vi "Close Private.vi"(8 "error in (no error)":errorcluster) -> (0 "error out":errorcluster)   [LabVIEW 2020, in "Better Search.lvlib" / "BetterSearch.lvclass"]
uses:
  BetterSearch.lvclass
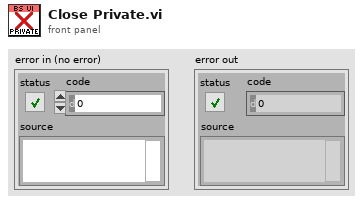
[diagram p1: front panel]
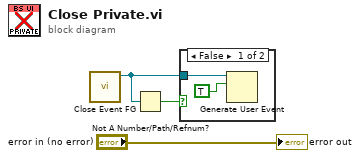
[diagram p0: block diagram]
diagram:
  n1 = call "Close Event FG.vi"() -> ("Close"=w1:refnum<user-event>)  [unwired: 11 in]
  n2 = Not A Number/Path/Refnum?(number/path/refnum=w1) -> (NaN/Path/Refnum?=w2:bool)
  n3 = case shown="False" w2 {
    tunnel: w1 -> [w5 _]
    frame False {
      n4 = Generate User Event(user event=w5, event data cluster=TRUE ("event data")) -> ()  [unwired: 2 in, 2 out]
    }
    frame True {
    }
  }
  "error out" <- "error in (no error)"
